vi "EthernetClient.vi"(7 "Port":u16=502, 8 "Address":string="127.0.0.1", 9 "Proto":i32(ring) items=["TCP", "UDP", "RTUOverTCP", "RTUOverUDP"]) -> (3 "Client":u64[](array[numeric]), 4 "error out":errorcluster)   [LabVIEW 2020, in "SnapMB.lvlib"]
uses:
  SnapMB.lvlib
  windows/snapmb.dll
panel:
  in  "error in":errorcluster
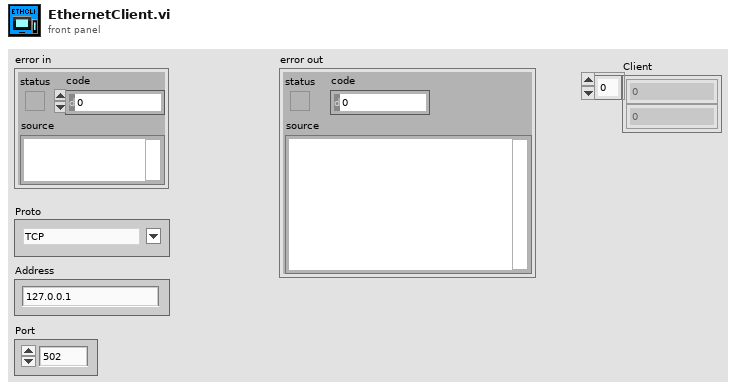
[diagram p1: front panel]
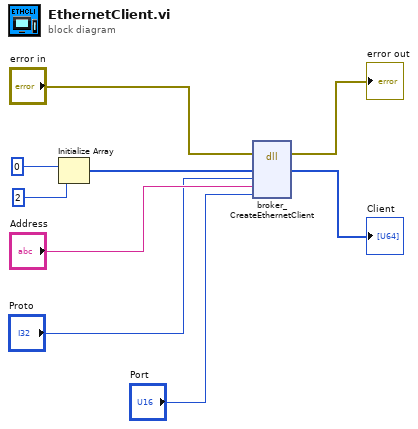
[diagram p0: block diagram]
diagram:
  n1 = Initialize Array(u64 0 ("element"), 2 ("dimension size")) -> (w3:u64[])
  n2 = dll-call lib="D:/SnapMB/LabView/lib/windows/snapmb.dll" fn="broker_CreateEthernetClient"(error in="error in", "Broker"=w3, "Proto"="Proto", "Address"="Address", "Port"="Port") -> (error out=→"error out":errorcluster, "Broker"=→"Client":u64[])  [unwired: 6 in, 1 out]
